vi "Draw BG Image.vi"(6 "Control Ref Queue":T4, 8 "error in (no error)":errorcluster, 10 "Multiplot Representation In":T1, 11 "2D Feather.lvclass in":refnum<class "2D Feather.lvclass">) -> (0 "error out":errorcluster, 2 "Multiplot Representation Out":T1, 3 "2D Feather.lvclass out":refnum<class "2D Feather.lvclass">)   [LabVIEW 2017, in "2D Feather.lvclass"]
uses:
  <vilib>/Math Plots/2D Math Plots/2D Feather/2D Feather/2D Feather.lvclass
  <vilib>/Math Plots/2D Math Plots/2D Plot/Action String/2DMathPlot Ctrl Act Queue.ctl
  <vilib>/Math Plots/2D Math Plots/2D Plot/Action String/2DMathPlot Ctrl Act Cluster.ctl
  <vilib>/Math Plots/2D Math Plots/2D Plot/Action String/2DMathPlot State Class.ctl
  e:/builds/penguin/labview/branches/2017/dev/dist/vi.lib/Math Plots/2D Math Plots/2D Plot/2D Plot/2D Plot.lvclass
  <vilib>/Math Plots/2D Math Plots/2D Plot/2D Plot/Typedef/Multiplot Representation.ctl
  <vilib>/Math Plots/2D Math Plots/2D Plot/2D Plot/Typedef/Plot Representation.ctl
  <vilib>/Math Plots/2D Math Plots/2D Plot/2D Plot/Typedef/Range Cluster.ctl
  <vilib>/Math Plots/2D Math Plots/2D Feather/2D Feather/2D Feather.lvclass/2D Feather.ctl
  <vilib>/Math Plots/2D Math Plots/2D Feather/2D Feather/Typedef/2D Feather Property.ctl
  <vilib>/Math Plots/2D Math Plots/2D Plot/2D Plot/2D Plot.lvclass
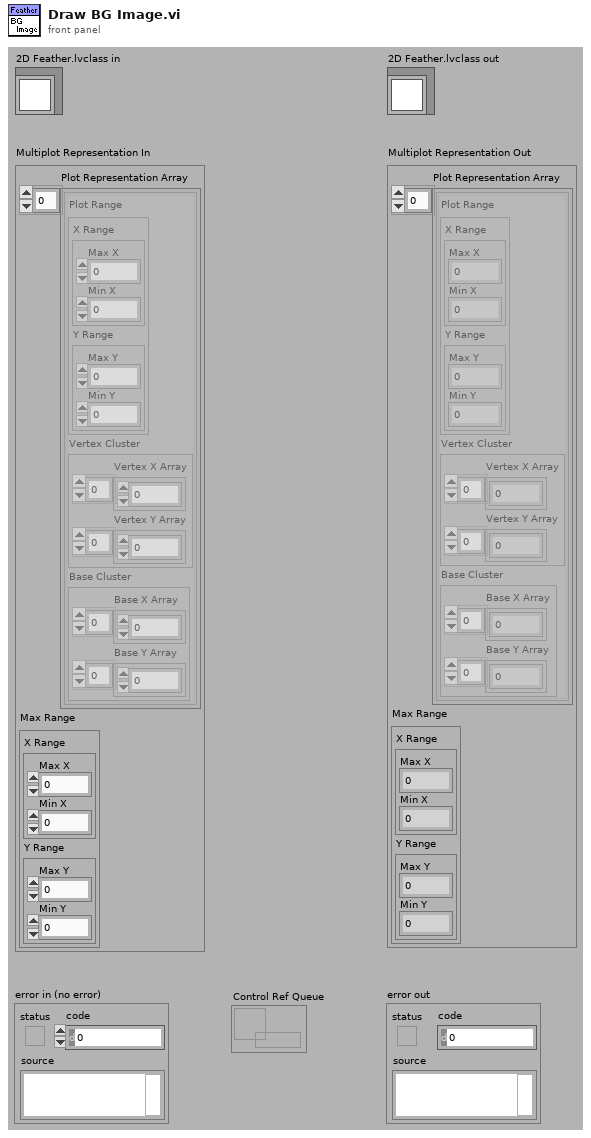
[diagram p1: front panel]
types:
  T1 = typedef "2D Plot.lvclass/Multiplot Representation.ctl" = cluster{"Plot Representation Array":T2[], "Max Range":T3}
  T2 = typedef "2D Plot.lvclass/Plot Representation.ctl" = cluster{"Plot Range":T3, "Vertex Cluster":cluster{"Vertex X Array":dbl[], "Vertex Y Array":dbl[]}, "Base Cluster":cluster{"Base X Array":dbl[], "Base Y Array":dbl[]}}
  T3 = typedef "2D Plot.lvclass/Range Cluster.ctl" = cluster{"X Range":cluster{"Max X":dbl, "Min X":dbl}, "Y Range":cluster{"Max Y":dbl, "Min Y":dbl}}
  T4 = typedef "2DMathPlot Ctrl Act Queue.ctl" = refnum<queue>
  T5 = typedef "2D Feather.lvclass/2D Feather Property Array.ctl" = T6[]
  T6 = typedef "2D Feather.lvclass/2D Feather Property.ctl" = cluster{"Arrow Size":dbl}
  T7 = typedef "2D Plot.lvclass/Plot Property Array.ctl" = T8[]
  T8 = typedef "2D Plot.lvclass/Plot Property.ctl" = cluster{"Bar Plot Style":u8, "DigitalLineStyle":u8, "TransitionLocation":u8, "Transition Type":u8, "Fill To":i16, "Fill/Pt. Color":u32, "Label Style":u8, "Line Style":u8, "Line Width":u8, "Plot Color":u32, "Plot Interpolation":u8, "Plot Name":string, "Point Style":u8, "Visible?":bool, "XScaleIdx":u32, "YScaleIdx":u32}
  T9 = typedef "2DMathPlot Ctrl Act Cluster.ctl" = cluster{"Plot Area Ref":refnum<vi>, "Z Axis Ref":refnum<vi>, "Legend Ref":refnum<vi>, "XControl Ref":refnum<vi>, "Facade Ref":refnum<vi>, "Display State Change Class":T10}
  T10 = typedef "2DMathPlot State Class.ctl" = enum16{"Update All (Undo)", "Update General", "Update Appearance", "Update Format", "Update Scale", "Update Marker", "Update Cursor", "None"}
  T11 = cluster{"Width":u16, "Style":enum32{"Solid", "Dash", "Dot", "DashDot", "DashDotDot"}}
  T12 = cluster{"Base X Array":dbl[], "Base Y Array":dbl[]}
  T13 = cluster{"Vertex X Array":dbl[], "Vertex Y Array":dbl[]}
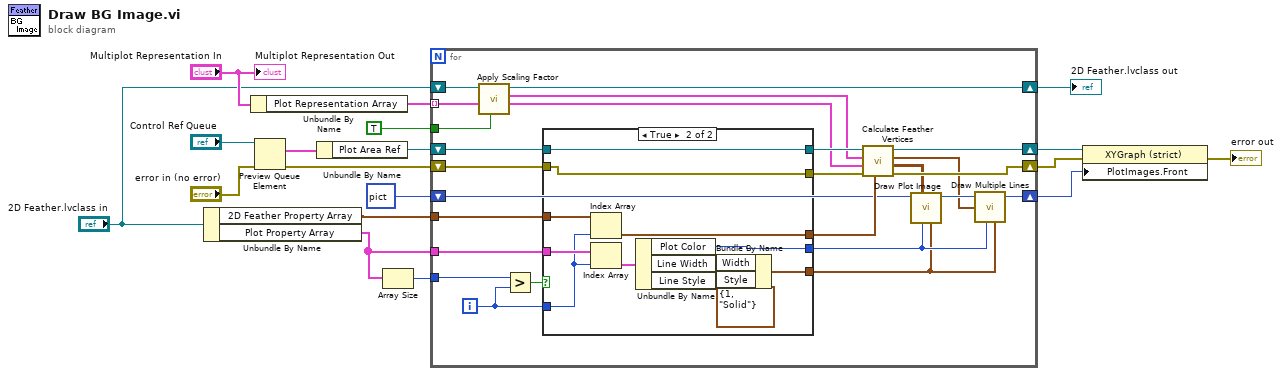
[diagram p0: block diagram]
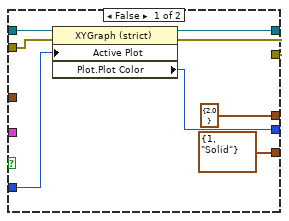
[diagram p2: hidden frame]
diagram:
  n1 = Unbundle By Name("2D Feather.lvclass in") -> ("2D Feather Property Array"=w14:T5, "Plot Property Array"=w5:T7)
  n2 = Unbundle By Name("Multiplot Representation In") -> ("Plot Representation Array"=w11:T2[])
  n3 = Preview Queue Element(queue="Control Ref Queue", error in (no error)="error in (no error)") -> (element=w10:T9, error out=w17:errorcluster)  [unwired: 3 out]
  n4 = Unbundle By Name(w10) -> ("Plot Area Ref"=w15:refnum<vi>)
  n5 = Array Size(array=w5) -> (size(s)=w4:i32)
  n6 = for {
    tunnel: w11 -> [w24] mode=indexing
    shift-right: [w35] -> w13
    shift-left: picture data[5B] ("Picture In") -> [w38]
    tunnel: w5 -> [w43]
    tunnel: w14 -> [w42]
    shift-right: [w40] -> w16
    shift-left: w15 -> [w28]
    shift-right: [w39] -> w18
    shift-left: w17 -> [w26]
    tunnel: w4 -> [w31]
    tunnel: TRUE ("Apply to Vertex?") -> [w21]
    shift-right: [w19] -> w1
    shift-left: "2D Feather.lvclass in" -> [w20]
    i -> [w30]
    n7 = call <vilib>:"Apply Scaling Factor.vi"("Apply to Vertex?"=w21, "Plot Representation Cluster"=w24, "2D Plot.lvclass in"=w20) -> ("Base Cluster"=w22:T12, "Vertex Cluster"=w23:T13, "2D Plot.lvclass out"=w19:refnum<class "2D Feather.lvclass">)  [unwired: 1 in, 5 out]
    n8 = Greater?(x=w31, y=w30) -> (0:w29:bool)
    n9 = case shown="True" w29 {
      tunnel: w43 -> [_ w63]
      tunnel: w42 -> [_ w62]
      tunnel: [T6 {"Arrow Size"=2.0} ("2D Feather Property") w61] -> w41
      tunnel: [w44 w56] -> w33
      tunnel: [T11 {"Width"=1, "Style"=enum."Solid"} ("pen") w55] -> w32
      tunnel: w30 -> [w45 w54]
      tunnel: w28 -> [w49 w52]
      tunnel: [w48 w52] -> w27
      tunnel: w26 -> [w47 w53]
      tunnel: [w46 w53] -> w25
      frame False {
        n10 = property class="XYGraph (strict)"(reference=w49, error in=w47, "Active Plot"=w45) -> (reference out=w48:refnum<vi>, error out=w46:errorcluster, "Plot.Plot Color"=w44:u32)
      }
      frame True {
        n11 = Index Array(array=w62, index=w54) -> (element=w61:T6)
        n12 = Index Array(array=w63, index=w54) -> (element=w57:T8)
        n13 = Unbundle By Name(w57) -> ("Plot Color"=w56:u32, "Line Width"=w59:u8, "Line Style"=w58:u8)
        n14 = Bundle By Name(cluster=T11 {"Width"=1, "Style"=enum."Solid"} ("pen"), "Width"=w59, "Style"=w58) -> (w55:T11)
      }
    }
    n15 = call <vilib>:"Calculate Feather Vertices.vi"("2D Feather Property"=w41, "error in (no error)"=w25, "Base Cluster"=w22, "Vertex Cluster"=w23, "Plot Area Ref"=w27) -> ("error out"=w39:errorcluster, "Feather Vertex"=w37:cluster{"X":i16, "Y":i16}[][], "Center Line Vertex"=w34:cluster{"X":i16, "Y":i16}[], "Dup Plot Area Ref"=w40:refnum<vi>)  [unwired: 3 out]
    n16 = call <vilib>:"Draw Plot Image.vi"("pen"=w32, "Plot Color"=w33, "Plot Vertex"=w37, "Picture In"=w38) -> ("Picture Out"=w36:picture)  [unwired: 7 out]
    n17 = call <vilib>:"Draw Multiple Lines.vi"("picture"=w36, "line endpoints"=w34, "color(black)"=w33, "pen"=w32) -> ("new picture"=w35:picture)  [unwired: 1 in, 4 out]
  }
  "2D Feather.lvclass out" <- w1
  n18 = property class="XYGraph (strict)"(reference=w16, error in=w18, "PlotImages.Front"=w13) -> (error out=→"error out":errorcluster)  [unwired: 1 out]
  "Multiplot Representation Out" <- "Multiplot Representation In"
